vi "Log.vi"(8 "error in (no error)":errorcluster, 9 "Timestamp data points":bool, 10 "tdms file":refnum<k34>, 11 "Acquired Result in":refnum<class "Acquired Result.lvclass">) -> (0 "error out":errorcluster, 2 "tdms file out":refnum<k34>, 3 "Acquired Result out":refnum<class "Acquired Result.lvclass">)   [LabVIEW 2016, in "Acquired Result.lvclass"]
uses:
  Acquired Result.lvclass
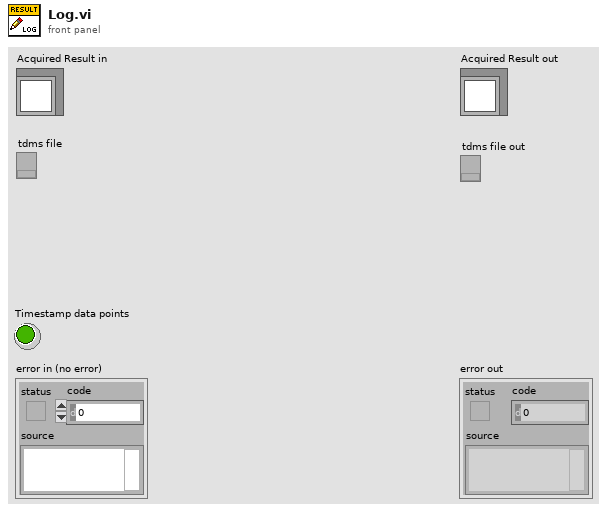
[diagram p1: front panel]
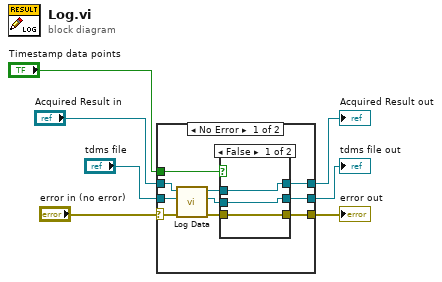
[diagram p0: block diagram]
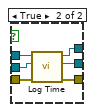
[diagram p2: hidden frame]
diagram:
  n1 = case shown="No Error" "error in (no error)" {
    selector: "error in (no error)" -> [w13 w27]
    tunnel: "Acquired Result in" -> [w10 w29]
    tunnel: "tdms file" -> [w16 w28]
    tunnel: [w14 w28] -> w5
    tunnel: [w9 w29] -> w4
    tunnel: [w12 w27] -> w3
    tunnel: "Timestamp data points" -> [w8 _]
    frame No Error {
      n2 = call-dynamic "Log Data.vi"("error in (no error)"=w13, "tdms file"=w16, "Acquired Result in"=w10) -> ("error out"=w17:errorcluster, "tdms file out"=w15:refnum<k34>, "Acquired Result out"=w11:refnum<class "Acquired Result.lvclass">)  [unwired: 6 in]
      n3 = case shown="False" w8 {
        tunnel: w17 -> [w18 w26]
        tunnel: w15 -> [w19 w25]
        tunnel: [w19 w24] -> w14
        tunnel: [w18 w23] -> w12
        tunnel: w11 -> [w20 w22]
        tunnel: [w20 w21] -> w9
        frame False {
        }
        frame True {
          n4 = call-dynamic "Log Time.vi"("error in (no error)"=w26, "tdms file"=w25, "Acquired Result in"=w22) -> ("error out"=w23:errorcluster, "tdms file out"=w24:refnum<k34>, "Acquired Result out"=w21:refnum<class "Acquired Result.lvclass">)  [unwired: 6 in]
        }
      }
    }
    frame Error {
    }
  }
  "error out" <- w3
  "Acquired Result out" <- w4
  "tdms file out" <- w5
